vi "extract PLC raw to actual.vi"(10 "Raw data":string, 11 "Enum":T1(ring)=enum."Data Register(D)") -> (2 "M":bool[](array[boolean]), 3 "Analog":dbl[](array[numeric]))   [LabVIEW 2015]
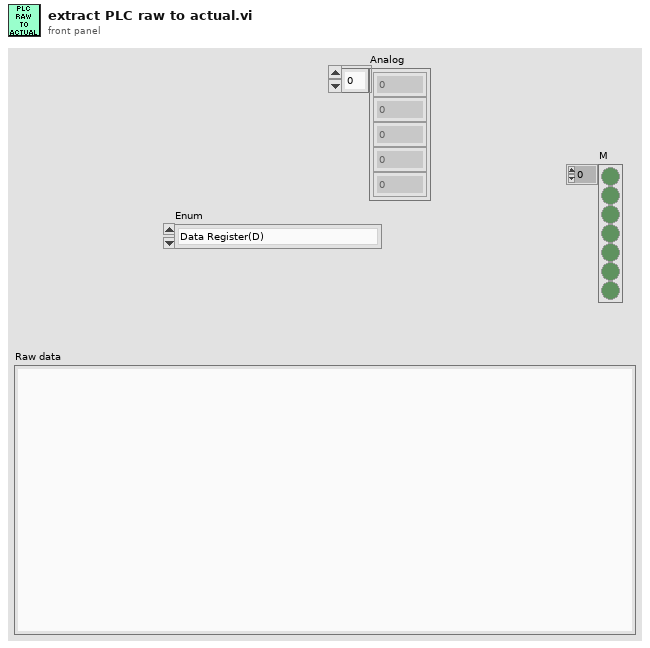
[diagram p1: front panel]
types:
  T1 = enum16{"Input(X)", "Output(Y)", "internal relay(M)", "Data Register(D)"}
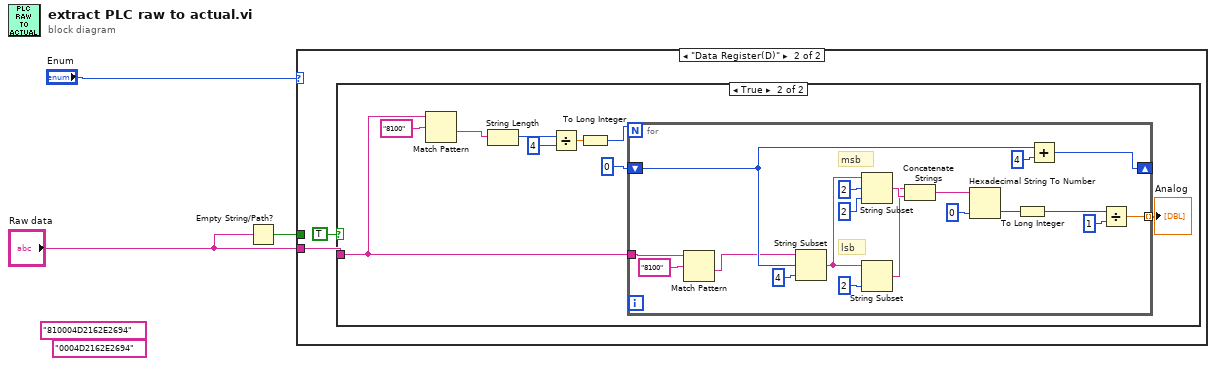
[diagram p0: block diagram]
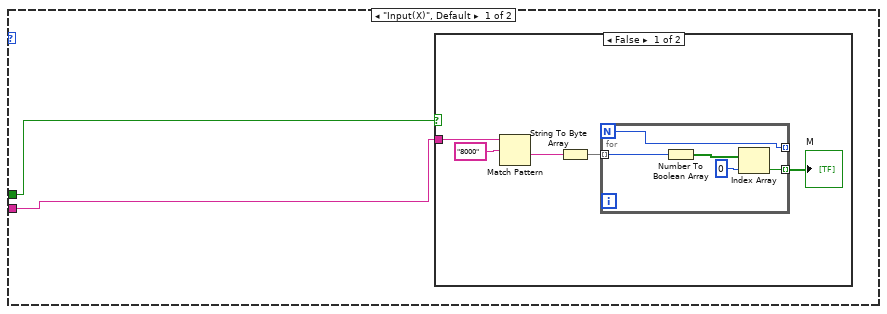
[diagram p2: hidden frame]
diagram:
  (unwired) "0004D2162E2694" ("String")
  (unwired) "810004D2162E2694" ("Raw data 2")
  n1 = Empty String/Path?(string/path="Raw data") -> (empty?=w1:bool)
  n2 = case shown="\"Data Register(D)\"" "Enum" {
    tunnel: "Raw data" -> [w5 w17]
    tunnel: w1 -> [w4 _]
    frame "Input(X)", Default {
      n3 = case shown="False" w4 {
        tunnel: w5 -> [w9 _]
        frame False {
          n4 = Match Pattern(string=w9, regular expression="8000") -> (after substring=w7:string)  [unwired: 1 in, 3 out]
          n5 = String To Byte Array(string=w7) -> (unsigned byte array=w8:u8[])
          n6 = for {
            N -> [w13]
            tunnel: w8 -> [w15] mode=indexing
            tunnel: [w13] -> _ mode=indexing
            tunnel: [w11] -> w6 mode=indexing
            n7 = Number To Boolean Array(number=w15) -> (Boolean array=w14:bool[])
            n8 = Index Array(array=w14, index=0) -> (element=w11:bool)
          }
          "M" <- w6
        }
        frame True {
        }
      }
    }
    frame "Data Register(D)" {
      n9 = case shown="True" TRUE {
        tunnel: w17 -> [_ w24]
        frame False {
        }
        frame True {
          n10 = Match Pattern(string=w24, regular expression="8100") -> (after substring=w23:string)  [unwired: 1 in, 3 out]
          n11 = String Length(string=w23) -> (length=w22:i32)
          n12 = Divide(x=w22, y=4) -> (x/y=w20:dbl)
          n13 = To Long Integer(number=w20) -> (32bit integer=w18:i32)
          n14 = for {
            N: w18 -> [_]
            shift-right: [w45] -> _
            shift-left: 0 -> [w43]
            tunnel: w24 -> [w28]
            tunnel: [w30] -> w19 mode=indexing
            # "lsb"
            # "msb"
            n15 = Match Pattern(string=w28, regular expression="8100") -> (after substring=w27:string)  [unwired: 1 in, 3 out]
            n16 = String Subset(string=w27, offset (0)=w43, length (rest)=4 ("length (rest)")) -> (substring=w38:string)
            n17 = String Subset(string=w38, offset (0)=2, length (rest)=2 ("length (rest)")) -> (substring=w37:string)
            n18 = String Subset(string=w38, length (rest)=2 ("length (rest)")) -> (substring=w36:string)  [unwired: 1 in]
            n19 = Concatenate Strings(w36, w37) -> (w35:string)
            n20 = Hexadecimal String To Number(string=w35, default (0uL)=u32 0 ("default (0 U32)")) -> (number=w31:u32)  [unwired: 1 in, 1 out]
            n21 = To Long Integer(number=w31) -> (32bit integer=w32:i32)
            n22 = Add(x=w43, y=4) -> (x+y=w45:i32)
            n23 = Divide(x=w32, y=u32 1) -> (x/y=w30:dbl)
          }
          "Analog" <- w19
        }
      }
    }
  }
